vi "Get Refnum Type Enum from TD__ogtk.vi"(4 "Type Descriptor":T1) -> (1 "Refnum Subtype Enum":T2 format="%.0x")   [LabVIEW 2020]
doc: "Gets a Refnum Subtype Enumeration from a Type Descriptor Array."
uses:
  <userlib>/_OpenG.lib/lvdata/lvdata.llb/Refnum Subtype Enum__ogtk.ctl
  <userlib>/_OpenG.lib/lvdata/lvdata.llb/Type Descriptor__ogtk.ctl
panel:
  # "Please visit http://www.OpenG.org to learn about the\nOpen Source LabVIEW software movement.\n\nNOTICE -- YOU MUST LEAVE THIS NOTICE IN PLACE.  PER THE TERMS OF THE LICENSE BELOW, YOU MAY SUBLICENSE THIS SOFTWARE \nIN ANY WAY THAT DOES NOT CONFLICT WITH THIS LICENSE.\n\n### BSD License (http://www.opensource.org/licenses/bsd-license.php) Begin ###\n \nCopyright (c) 2002-2011, Jim Kring <jim@jimkring.com>\nCopyright (c) 2011, Jonathon Green <jg@jgcode.net>\n\nAll rights reserved.\n\nRedistribution and use in source and binary forms, with or without modification, are permitted provided that the following conditions are met:\n\n    * Redistributions of source code must retain the above copyright notice, this list of conditions and the following disclaimer.\n    * Redistributions in binary form must reproduce the above copyright notice, this list of conditions and the following disclaimer in the \n       documentation and/or other materials provided with the distribution.\n    * Neither the name of SciWare, James Kring, Inc., nor the names of its contributors may be used to endorse or promote products derived \n       from this software without specific prior written permission.\n\nTHIS SOFTWARE IS PROVIDED BY THE COPYRIGHT HOLDERS AND CONTRIBUTORS \"AS IS\" AND ANY EXPRESS OR IMPLIED WARRANTIES, \nINCLUDING, BUT NOT LIMITED TO, THE IMPLIED WARRANTIES OF MERCHANTABILITY AND FITNESS FOR A PARTICULAR PURPOSE ARE \nDISCLAIMED. IN NO EVENT SHALL THE COPYRIGHT OWNER OR CONTRIBUTORS BE LIABLE FOR ANY DIRECT, INDIRECT, INCIDENTAL,\n SPECIAL, EXEMPLARY, OR CONSEQUENTIAL DAMAGES (INCLUDING, BUT NOT LIMITED TO, PROCUREMENT OF SUBSTITUTE GOODS OR \nSERVICES; LOSS OF USE, DATA, OR PROFITS; OR BUSINESS INTERRUPTION) HOWEVER CAUSED AND ON ANY THEORY OF LIABILITY, \nWHETHER IN CONTRACT, STRICT LIABILITY, OR TORT (INCLUDING NEGLIGENCE OR OTHERWISE) ARISING IN ANY WAY OUT OF THE USE \nOF THIS SOFTWARE, EVEN IF ADVISED OF THE POSSIBILITY OF SUCH DAMAGE.\n\n### BSD License End ###"
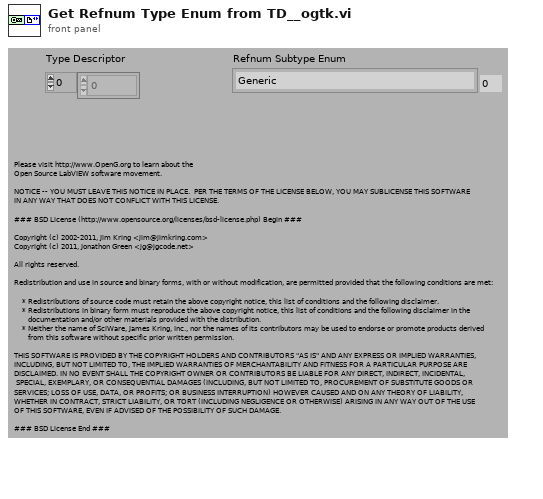
[diagram p1: front panel]
types:
  T1 = typedef "Type Descriptor__ogtk.ctl" = i16[]
  T2 = typedef "Refnum Subtype Enum__ogtk.ctl" = enum8{"Generic", "Datalog File Refnum", "Byte Stream File Refnum", "Device Refnum", "Occurence Refnum", "TCP Connection Refnum", "VISA Refnum (Obsolete)", "Automation Renum", "VI Server Refnum", "Menu Refnum", "IVI Refnum (Obsolete)", "IMAQ Session", "0x0C", "Datasocket Refnum", "VISA Resource", "IVI Logical Name", "UDP Connection Refnum", "Notifier Refnum", "Queue Refnum", "IrDA Refnum", "Hardware Plugin Refnum", "Hardware Plugin Tag Refnum", "DAQmx Refnum", "Event Registration Refnum", ".NET Refnum", "User Event Refnum", "0x1A", "Event Callback", "0x1C", "0x1D", "LabVIEW Class Instance", "Bluetooth", "Data Value References", "RT FIFO", "TDM Streaming"}
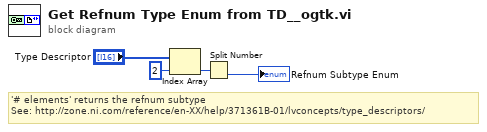
[diagram p0: block diagram]
diagram:
  # "'# elements' returns the refnum subtype\nSee: http://zone.ni.com/reference/en-XX/help/371361B-01/lvconcepts/type_descriptors/"
  n1 = Index Array(array="Type Descriptor", index=2) -> (element=w2:i16)
  n2 = Split Number(x=w2) -> (lo(x)=→"Refnum Subtype Enum":u8)  [unwired: 1 out]
